vi "Get All Sequence Error Messages.vi"(8 "error in (no error)":errorcluster, 11 "Variant in":variant) -> (0 "error out":errorcluster, 1 "TSA Errors as Plain Text":string, 2 "TSA Errors[]":T1[](array[typedef]), 3 "Variant out":variant)   [LabVIEW 2016, in "SLL TestStand.lvlib"]
uses:
  SLL TestStand.lvlib
  _Typedefs/TSA Error Message Cluster.ctl
  SLL String/_SubVIs/1D String Array to String.vi
  SLL String/SLL String.lvlib
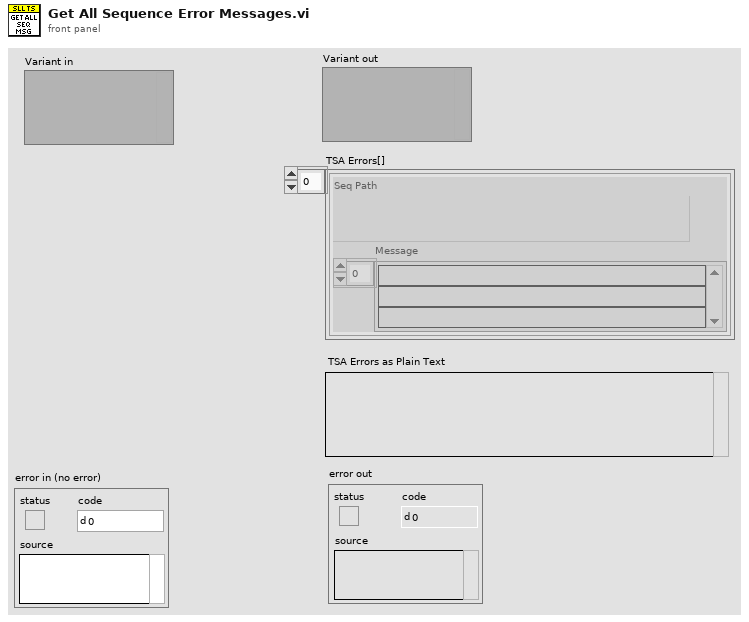
[diagram p1: front panel]
types:
  T1 = typedef "SLL TestStand.lvlib/TSA Error Message Cluster.ctl" = cluster{"Seq Path":path, "Message":string[]}
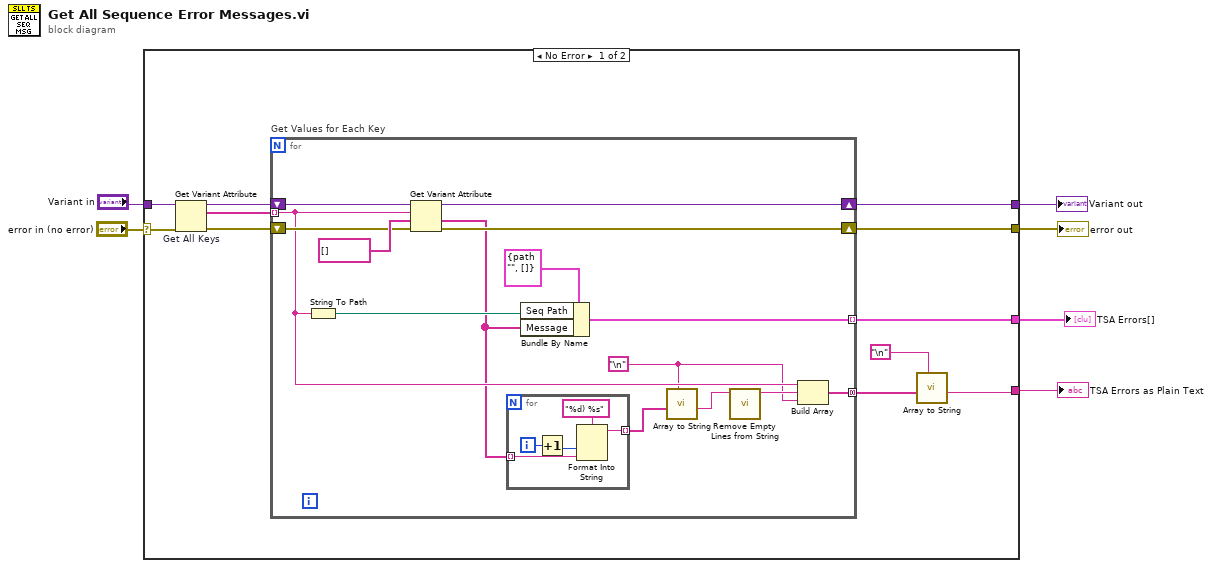
[diagram p0: block diagram]
diagram:
  n1 = case shown="No Error" "error in (no error)" {
    selector: "error in (no error)" -> [w12 w39]
    tunnel: "Variant in" -> [w17 w38]
    tunnel: [w13 w38] -> w5
    tunnel: [w11 w39] -> w3
    tunnel: [w10 _] -> w2
    tunnel: [w7 _] -> w1
    frame No Error {
      n2 = Get Variant Attribute "Get All Keys"(Variant=w17, error in=w12) -> (duplicate Variant=w16:variant, names=w15:string[], error out=w14:errorcluster)  [unwired: 2 in, 1 out]
      n3 = for "Get Values for Each Key" {
        shift-right: [w31] -> w13
        shift-left: w16 -> [w32]
        tunnel: w15 -> [w23] mode=indexing
        shift-right: [w28] -> w11
        shift-left: w14 -> [w29]
        tunnel: [w25] -> w10 mode=indexing
        tunnel: [w21] -> w9 mode=concatenating
        w18 = "\n"
        n4 = String To Path(string=w23) -> (path=w26:path)
        n5 = Get Variant Attribute(Variant=w32, name=w23, default value (empty Variant)=string[] [], error in=w29) -> (duplicate Variant=w31:variant, value=w20:string[], error out=w28:errorcluster)  [unwired: 1 out]
        n6 = for {
          tunnel: w20 -> [w35] mode=indexing
          tunnel: [w34] -> w19 mode=indexing
          i -> [w37]
          n7 = Increment(x=w37) -> (x+1=w33:i32)
          n8 = Format Into String(format string="%d) %s", w33, w35) -> (resulting string=w34:string)  [unwired: 2 in, 1 out]
        }
        n9 = Bundle By Name(cluster=T1 {"Seq Path"=path "", "Message"=[]} ("TSA Message"), "Seq Path"=w26, "Message"=w20) -> (w25:T1)
        n10 = call-poly "Array to String.vi"("Delimiter (,)"=w18, "1D Array[]"=w19) -> ("String"=w24:string)  [unwired: 6 in]
        n11 = call "Remove Empty Lines from String.vi"("String"=w24) -> ("String Out"=w22:string)  [unwired: 10 in]
        n12 = Build Array(w23, w22, w18) -> (w21:string[])
      }
      n13 = call-poly "Array to String.vi"("Delimiter (,)"="\n", "1D Array[]"=w9) -> ("String"=w7:string)  [unwired: 6 in]
    }
    frame Error {
    }
  }
  "Variant out" <- w5
  "error out" <- w3
  "TSA Errors[]" <- w2
  "TSA Errors as Plain Text" <- w1
